vi "ActionVIOnLoad.vi"(8 "error in (no error)":errorcluster, 11 "Device Item Ref in":T1 format="%.0x") -> (0 "error out":errorcluster, 3 "Device Item Ref out":T1 format="%.0x")   [LabVIEW 2027, in "System Monitor System Explorer.lvlib"]
uses:
  System Monitor System Explorer.lvlib
  <vilib>/NI VeriStand/Custom Device API/Custom Device Item Ref.ctl
  <vilib>/NI VeriStand/Custom Device API/Custom Device API.lvlib
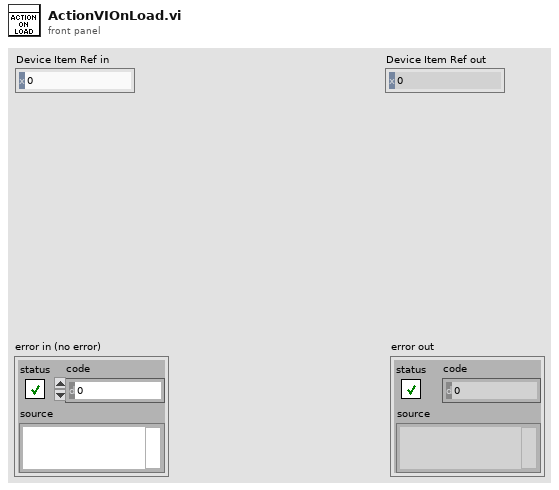
[diagram p1: front panel]
types:
  T1 = typedef "Custom Device API.lvlib/Custom Device Item Ref.ctl" = u64
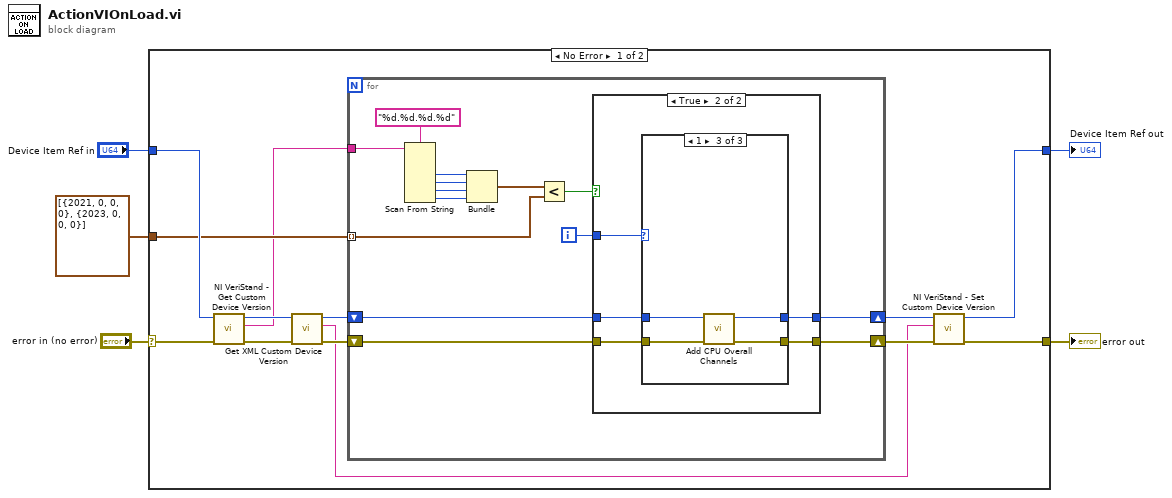
[diagram p0: block diagram]
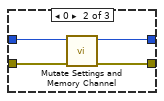
[diagram p4: hidden frame]
diagram:
  n1 = case shown="No Error" "error in (no error)" {
    selector: "error in (no error)" -> [w18 w51]
    tunnel: [w15 w51] -> w3
    tunnel: [w16 w50] -> w2
    tunnel: "Device Item Ref in" -> [w17 w50]
    tunnel: cluster{i32, i32, i32, i32}[] [{2021, 0, 0, 0}, {2023, 0, 0, 0}] -> [w14 _]
    frame No Error {
      n2 = call <vilib>:"NI VeriStand - Get Custom Device Version.vi"("error in (no error)"=w18, "Device Ref in"=w17) -> ("error out"=w9:errorcluster, "Value"=w6:string, "Device Ref out"=w11:T1)  [unwired: 7 in]
      n3 = call "Get XML Custom Device Version.vi"("error in (no error)"=w9, "Device Ref in"=w11) -> ("error out"=w8:errorcluster, "Version"=w7:string, "Device Ref out"=w10:T1)  [unwired: 7 in]
      n4 = for {
        tunnel: w6 -> [w30]
        tunnel: w14 -> [w29] mode=indexing
        shift-right: [w22] -> w13
        shift-left: w10 -> [w32]
        shift-right: [w21] -> w12
        shift-left: w8 -> [w31]
        i -> [w19]
        n5 = Scan From String(format string="%d.%d.%d.%d", input string=w30) -> (output 1=w27:i32, output 2=w26:i32, output 3=w25:i32, output 4=w24:i32)  [unwired: 6 in, 3 out]
        n6 = Bundle(w27, w26, w25, w24) -> (w23:cluster{i32, i32, i32, i32})  [unwired: 1 in]
        n7 = Less?(x=w23, y=w29) -> (x < y?=w20:bool)
        n8 = case shown="True" w20 {
          tunnel: w32 -> [w34 w39]
          tunnel: w31 -> [w33 w38]
          tunnel: [w34 w37] -> w22
          tunnel: [w33 w36] -> w21
          tunnel: w19 -> [_ w35]
          frame False {
          }
          frame True {
            n9 = case shown="1" w35 {
              tunnel: w39 -> [w41 w45 w47]
              tunnel: w38 -> [w40 w44 w49]
              tunnel: [w41 w43 w46] -> w37
              tunnel: [w40 w42 w48] -> w36
              frame Default {
              }
              frame 0 {
                n10 = call "Mutate Settings and Memory Channel.vi"("error in (no error)"=w44, "Item Ref in"=w45) -> ("error out"=w42:errorcluster, "Item Ref out"=w43:T1)  [unwired: 8 in]
              }
              frame 1 {
                n11 = call "Add CPU Overall Channels.vi"("error in"=w49, "custom device"=w47) -> ("error out"=w48:errorcluster, "custom device out"=w46:T1)  [unwired: 8 in]
              }
            }
          }
        }
      }
      n12 = call <vilib>:"NI VeriStand - Set Custom Device Version.vi"("error in (no error)"=w12, "Value"=w7, "Device Ref in"=w13) -> ("error out"=w15:errorcluster, "Device Ref out"=w16:T1)  [unwired: 7 in]
    }
    frame Error {
    }
  }
  "error out" <- w3
  "Device Item Ref out" <- w2
